vi "ROVFifoRead.vi"(11 "Cluster in":T1={"Connections"={"Ping1D - A"={"Connection"="", "error"={"status"=FALSE, "code"=0, "source"=""}, "Distance"=0.0, "FIFO"={"rt fifo"=refnum, "error"={"status"=FALSE, "code"=0, "source"=""}}}, "Ping1D - B"={"Connection"="", "error"={"status"=FALSE, "code"=0, "source"=""}, "Distance"=0.0, "FIFO"={"rt fifo"=refnum, "error"={"status"=FALSE, "code"=0, "source"=""}}}, "IMU"={"Error"={"status"=FALSE, "code"=0, "source"=""}, "FIFO"={"rt fifo"=refnum, "error"={"status"=FALSE, "code"=0, "source"=""}}}, "MotorControl"={"Rear"={"Error PWM"={"status"=FALSE, "code"=0, "source"=""}, "Error Direction"={"status"=FALSE, "code"=0, "source"=""}}, "Left"={"Error PWM"={"status"=FALSE, "code"=0, "source"=""}, "Error Direction"={"status"=FALSE, "code"=0, "source"=""}}, "Right"={"Error PWM"={"status"=FALSE, "code"=0, "source"=""}, "Error Direction"={"status"=FALSE, "code"=0, "source"=""}}}, "Bar100"={"I2C Ref Out"={"myRIO Reference"={"myRIO Model"=enum."Unknown", "myRIO Hardware Reference"={"Generic FPGA Reference"=refnum, "Allow multiple opens"=FALSE}}, "I2C Channels Enum"=enum."Not Connected", "I2C Configuration"={"I2C Transfer Rate"=enum."Fast mode (400 kbps)"}}, "error"={"status"=FALSE, "code"=0, "source"=""}, "Distance"=0.0, "FIFO"={"rt fifo"=refnum, "error"={"status"=FALSE, "code"=0, "source"=""}}}}, "sensorData"={"IMU Data"={"X-Axis"=0.0, "Y-Axis"=0.0, "Z-Axis"=0.0}, "Bar100 Data"={"Pressure"=0.0, "Temp"=0.0}}, "outputData"={"Rotation Angle"=0.0, "Rotation Vector"={"x"=0.0, "y"=0.0, "z"=0.0}, "PING A distance"=0.0, "Ping B distance"=0.0, "angles"={"roll"=0.0, "pitch"=0.0, "yaw"=0.0}}, "Writer"={"endpoint"="", "error"={"status"=FALSE, "code"=0, "source"=""}}, "PID"={"reinitialize?"=FALSE, "Depth"={"setpoint"=0.0, "Gains"={"proportional gain (Kc)"=1.0, "integral time (Ti, min)"=0.01, "derivative time (Td, min)"=0.0}}, "Roll"={"setpoint"=0.0, "Gains"={"proportional gain (Kc)"=1.0, "integral time (Ti, min)"=0.01, "derivative time (Td, min)"=0.0}}}} {"PID"."Roll"."setpoint" format="%.2f"; "PID"."Roll"."Gains"."derivative time (Td, min)" format="%.3f"; "PID"."Roll"."Gains"."integral time (Ti, min)" format="%.3f"; "PID"."Roll"."Gains"."proportional gain (Kc)" format="%.3f"; "PID"."Depth"."setpoint" format="%.2f"; "PID"."Depth"."Gains"."derivative time (Td, min)" format="%.3f"; "PID"."Depth"."Gains"."integral time (Ti, min)" format="%.3f"; "PID"."Depth"."Gains"."proportional gain (Kc)" format="%.3f"}) -> (2 "Connected":bool, 3 "Cluster out":T1={"Connections"={"Ping1D - A"={"Connection"="", "error"={"status"=FALSE, "code"=0, "source"=""}, "Distance"=0.0, "FIFO"={"rt fifo"=refnum, "error"={"status"=FALSE, "code"=0, "source"=""}}}, "Ping1D - B"={"Connection"="", "error"={"status"=FALSE, "code"=0, "source"=""}, "Distance"=0.0, "FIFO"={"rt fifo"=refnum, "error"={"status"=FALSE, "code"=0, "source"=""}}}, "IMU"={"Error"={"status"=FALSE, "code"=0, "source"=""}, "FIFO"={"rt fifo"=refnum, "error"={"status"=FALSE, "code"=0, "source"=""}}}, "MotorControl"={"Rear"={"Error PWM"={"status"=FALSE, "code"=0, "source"=""}, "Error Direction"={"status"=FALSE, "code"=0, "source"=""}}, "Left"={"Error PWM"={"status"=FALSE, "code"=0, "source"=""}, "Error Direction"={"status"=FALSE, "code"=0, "source"=""}}, "Right"={"Error PWM"={"status"=FALSE, "code"=0, "source"=""}, "Error Direction"={"status"=FALSE, "code"=0, "source"=""}}}, "Bar100"={"I2C Ref Out"={"myRIO Reference"={"myRIO Model"=enum."Unknown", "myRIO Hardware Reference"={"Generic FPGA Reference"=refnum, "Allow multiple opens"=FALSE}}, "I2C Channels Enum"=enum."Not Connected", "I2C Configuration"={"I2C Transfer Rate"=enum."Fast mode (400 kbps)"}}, "error"={"status"=FALSE, "code"=0, "source"=""}, "Distance"=0.0, "FIFO"={"rt fifo"=refnum, "error"={"status"=FALSE, "code"=0, "source"=""}}}}, "sensorData"={"IMU Data"={"X-Axis"=0.0, "Y-Axis"=0.0, "Z-Axis"=0.0}, "Bar100 Data"={"Pressure"=0.0, "Temp"=0.0}}, "outputData"={"Rotation Angle"=0.0, "Rotation Vector"={"x"=0.0, "y"=0.0, "z"=0.0}, "PING A distance"=0.0, "Ping B distance"=0.0, "angles"={"roll"=0.0, "pitch"=0.0, "yaw"=0.0}}, "Writer"={"endpoint"="", "error"={"status"=FALSE, "code"=0, "source"=""}}, "PID"={"reinitialize?"=FALSE, "Depth"={"setpoint"=0.0, "Gains"={"proportional gain (Kc)"=1.0, "integral time (Ti, min)"=0.01, "derivative time (Td, min)"=0.0}}, "Roll"={"setpoint"=0.0, "Gains"={"proportional gain (Kc)"=1.0, "integral time (Ti, min)"=0.01, "derivative time (Td, min)"=0.0}}}} {"PID"."Roll"."setpoint" format="%.2f"; "PID"."Roll"."Gains"."derivative time (Td, min)" format="%.3f"; "PID"."Roll"."Gains"."integral time (Ti, min)" format="%.3f"; "PID"."Roll"."Gains"."proportional gain (Kc)" format="%.3f"; "PID"."Depth"."setpoint" format="%.2f"; "PID"."Depth"."Gains"."derivative time (Td, min)" format="%.3f"; "PID"."Depth"."Gains"."integral time (Ti, min)" format="%.3f"; "PID"."Depth"."Gains"."proportional gain (Kc)" format="%.3f"})   [LabVIEW 2019]
uses:
  Connections.ctl
  ROVsensorData.ctl
  ROVdataOut.ctl
  ROVcluster.ctl
  <vilib>/myRIO/Common/Instrument Driver Framework/Utilities/typedefs/Hardware Version Enum.ctl
  <vilib>/myRIO/Common/Instrument Driver Framework/Utilities/typedefs/Generic FPGA Reference.ctl
  <vilib>/myRIO/Common/Instrument Driver Framework/Utilities/typedefs/myRIO v1.0 Reference.ctl
  <vilib>/myRIO/Common/Instrument Driver Framework/Utilities/typedefs/myRIO Generic Hardware Reference.ctl
  <vilib>/myRIO/Common/Instrument Driver Framework/myRIO v1.0/I2C/typedefs/I2C Channels Enum.ctl
  <vilib>/myRIO/Instrument Drivers/Onboard IO/I2C/typedefs/I2C Transfer Rate.ctl
  <vilib>/myRIO/Instrument Drivers/Onboard IO/I2C/I2C.lvlib
  <vilib>/myRIO/Instrument Drivers/Onboard IO/I2C/typedefs/I2C Configuration.ctl
  <vilib>/myRIO/Instrument Drivers/Onboard IO/I2C/typedefs/I2C Reference.ctl
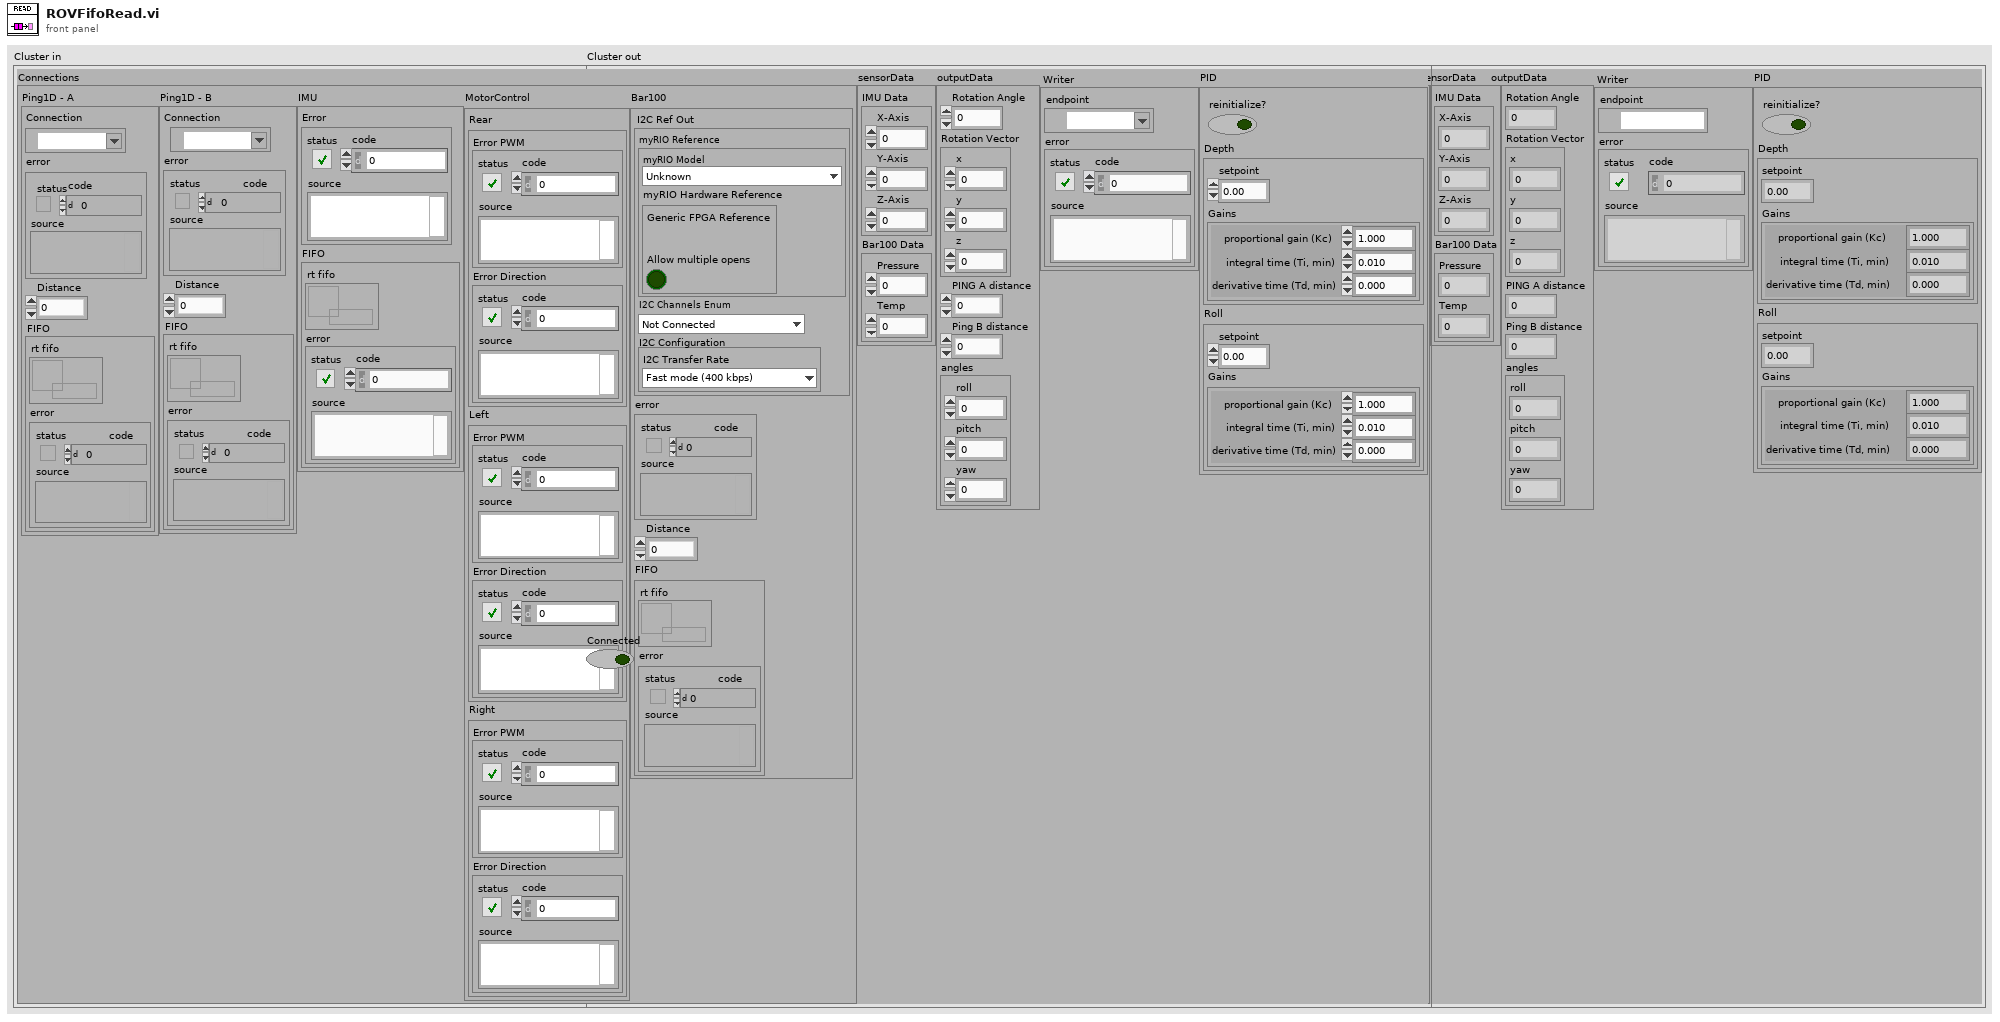
[diagram p1: front panel]
types:
  T1 = typedef "ROVcluster.ctl" = cluster{"Connections":T2, "sensorData":T11, "outputData":T12, "Writer":cluster{"endpoint":refnum<k21>, "error":errorcluster}, "PID":cluster{"reinitialize?":bool, "Depth":cluster{"setpoint":dbl, "Gains":cluster{"proportional gain (Kc)":dbl, "integral time (Ti, min)":dbl, "derivative time (Td, min)":dbl}}, "Roll":cluster{"setpoint":dbl, "Gains":cluster{"proportional gain (Kc)":dbl, "integral time (Ti, min)":dbl, "derivative time (Td, min)":dbl}}}}
  T2 = typedef "Connections.ctl" = cluster{"Ping1D - A":cluster{"Connection":refnum<visa-resource-name>, "error":errorcluster, "Distance":dbl, "FIFO":cluster{"rt fifo":refnum<k33>, "error":errorcluster}}, "Ping1D - B":cluster{"Connection":refnum<visa-resource-name>, "error":errorcluster, "Distance":dbl, "FIFO":cluster{"rt fifo":refnum<k33>, "error":errorcluster}}, "IMU":cluster{"Error":errorcluster, "FIFO":cluster{"rt fifo":refnum<k33>, "error":errorcluster}}, "MotorControl":cluster{"Rear":cluster{"Error PWM":errorcluster, "Error Direction":errorcluster}, "Left":cluster{"Error PWM":errorcluster, "Error Direction":errorcluster}, "Right":cluster{"Error PWM":errorcluster, "Error Direction":errorcluster}}, "Bar100":cluster{"I2C Ref Out":T3, "error":errorcluster, "Distance":dbl, "FIFO":cluster{"rt fifo":refnum<k33>, "error":errorcluster}}}
  T3 = typedef "I2C.lvlib/I2C Reference.ctl" = cluster{"myRIO Reference":T4, "I2C Channels Enum":T8, "I2C Configuration":T9}
  T4 = typedef "myRIO Generic Hardware Reference.ctl" = cluster{"myRIO Model":T5, "myRIO Hardware Reference":T6}
  T5 = typedef "Hardware Version Enum.ctl" = enum16{"Unknown", "myRIO-1900", "myRIO-1950", "roboRIO", "NI ELVIS RIO CM", "ELVIS III"}
  T6 = typedef "myRIO v1.0 Reference.ctl" = cluster{"Generic FPGA Reference":T7, "Allow multiple opens":bool}
  T7 = typedef "Generic FPGA Reference.ctl" = refnum<k20>
  T8 = typedef "I2C Channels Enum.ctl" = enum16{"Not Connected", "A/I2C", "B/I2C", "I2C/I2C"}
  T9 = typedef "I2C.lvlib/I2C Configuration.ctl" = cluster{"I2C Transfer Rate":T10}
  T10 = typedef "I2C.lvlib/I2C Transfer Rate.ctl" = enum16{"Standard mode (100 kbps)", "Fast mode (400 kbps)"}
  T11 = typedef "ROVsensorData.ctl" = cluster{"IMU Data":cluster{"X-Axis":dbl, "Y-Axis":dbl, "Z-Axis":dbl}, "Bar100 Data":cluster{"Pressure":dbl, "Temp":dbl}}
  T12 = typedef "ROVdataOut.ctl" = cluster{"Rotation Angle":dbl, "Rotation Vector":cluster{"x":dbl, "y":dbl, "z":dbl}, "PING A distance":dbl, "Ping B distance":dbl, "angles":cluster{"roll":dbl, "pitch":dbl, "yaw":dbl}}
  T13 = cluster{"X-Axis":dbl, "Y-Axis":dbl, "Z-Axis":dbl}
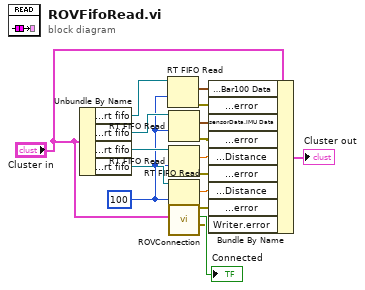
[diagram p0: block diagram]
diagram:
  w4 = 100 ("timeout in ms (0)")
  n1 = Unbundle By Name("Cluster in") -> ("Connections.Bar100.FIFO.rt fifo"=w2:refnum<k33>, "Connections.IMU.FIFO.rt fifo"=w14:refnum<k33>, "Connections.Ping1D - A.FIFO.rt fifo"=w11:refnum<k33>, "Connections.Ping1D - B.FIFO.rt fifo"=w10:refnum<k33>)
  n2 = RT FIFO Read(0:w2, 2:w4) -> (9:w1:cluster{"Pressure":dbl, "Temp":dbl}, 11:w3:errorcluster)  [unwired: 2 in, 3 out]
  n3 = RT FIFO Read(0:w14, 2:w4) -> (9:w16:T13, 11:w12:errorcluster)  [unwired: 2 in, 3 out]
  n4 = RT FIFO Read(0:w11, 2:w4) -> (9:w7:dbl, 11:w9:errorcluster)  [unwired: 2 in, 3 out]
  n5 = RT FIFO Read(0:w10, 2:w4) -> (9:w6:dbl, 11:w8:errorcluster)  [unwired: 2 in, 3 out]
  n6 = call "ROVConnection.vi"("Cluster in"="Cluster in") -> ("error out"=w5:errorcluster, "Connected"=→"Connected":bool)  [unwired: 9 in]
  n7 = Bundle By Name(cluster="Cluster in", "sensorData.Bar100 Data"=w1, "Connections.Bar100.FIFO.error"=w3, "sensorData.IMU Data"=w16, "Connections.IMU.FIFO.error"=w12, "Connections.Ping1D - A.Distance"=w7, "Connections.Ping1D - A.FIFO.error"=w9, "Connections.Ping1D - B.Distance"=w6, "Connections.Ping1D - B.FIFO.error"=w8, "Writer.error"=w5) -> (→"Cluster out":T1)
